vi "Write Memory Test Results.vi"(6 "Position":u32, 9 "error in (no error)":errorcluster, 10 "Read Passed":bool, 11 "Write Passed":bool) -> ()   [LabVIEW 2015, in "MTS Memory Test.lvclass"]
uses:
  MTS Memory Test.lvclass
  <vilib>/Cree, Inc/Cree Test Framework/Core Launcher/Core Manager Methods -- Enum.ctl
  <vilib>/Cree, Inc/Cree Test Framework/Core Launcher/Core Launcher.lvlib
  <vilib>/Cree, Inc/Cree Test Framework/Classes/Data/Data Repo/Class/Data Repo.lvclass
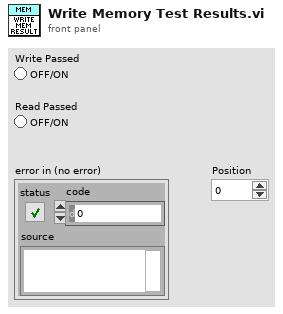
[diagram p1: front panel]
types:
  T1 = typedef "Core Launcher.lvlib/Core Manager Methods -- Enum.ctl" = enum16{"Spawn Objects", "Get Objects", "Destroy Objects"}
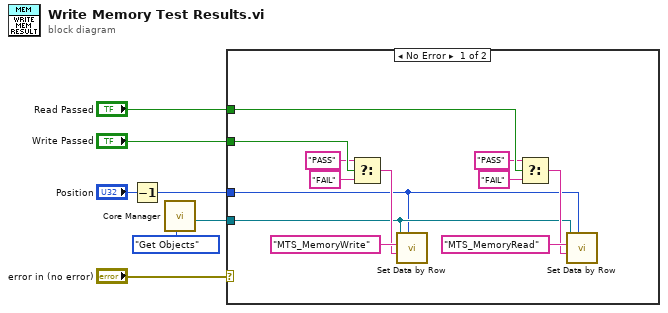
[diagram p0: block diagram]
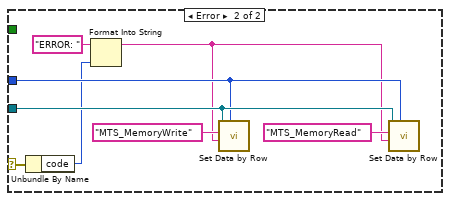
[diagram p2: hidden frame]
diagram:
  n1 = Decrement(x="Position") -> (x-1=w7:u32)
  n2 = call <vilib>:"Core Manager.vi"("Method"=Core_Manager_Methods_--_Enum."Get Objects") -> ("Data Repo"=w4:refnum<class "Data Repo.lvclass">)  [unwired: 6 in, 4 out]
  n3 = case shown="No Error" "error in (no error)" {
    selector: "error in (no error)" -> [_ w22]
    tunnel: "Write Passed" -> [w19 _]
    tunnel: "Read Passed" -> [w18 _]
    tunnel: w4 -> [w9 w25]
    tunnel: w7 -> [w8 w24]
    frame No Error {
      n4 = Select(t="PASS" ("Header"), s=w19, f="FAIL" ("Header")) -> (s? t:f=w14:string)
      n5 = call <vilib>:"Set Data by Row.vi"("Row"=w8, "Value"=w14, "Header"="MTS_MemoryWrite", "Acrobat Template in"=w9) -> ()  [unwired: 6 in, 2 out]
      n6 = Select(t="PASS" ("Header"), s=w18, f="FAIL" ("Header")) -> (s? t:f=w10:string)
      n7 = call <vilib>:"Set Data by Row.vi"("Row"=w8, "Value"=w10, "Header"="MTS_MemoryRead", "Acrobat Template in"=w9) -> ()  [unwired: 6 in, 2 out]
    }
    frame Error {
      n8 = Unbundle By Name(w22) -> ("code"=w21:i32)
      n9 = Format Into String(initial string="ERROR: " ("Header"), w21) -> (resulting string=w20:string)  [unwired: 2 in, 1 out]
      n10 = call <vilib>:"Set Data by Row.vi"("Row"=w24, "Value"=w20, "Header"="MTS_MemoryWrite", "Acrobat Template in"=w25) -> ()  [unwired: 6 in, 2 out]
      n11 = call <vilib>:"Set Data by Row.vi"("Row"=w24, "Value"=w20, "Header"="MTS_MemoryRead", "Acrobat Template in"=w25) -> ()  [unwired: 6 in, 2 out]
    }
  }
